vi "PICT_to_CAM.vi"(4 "Pict Refnum":refnum<vi>, 5 "IntGraph Refnum":refnum<vi>, 6 "Ny":i32, 7 "Yo":i32, 8 "Nx":i32, 9 "Xo":i32) -> (0 "Ny CAM":i16, 1 "Nx CAM":i16, 2 "Yo CAM":i16, 3 "Xo CAM":i16)   [LabVIEW 2011]
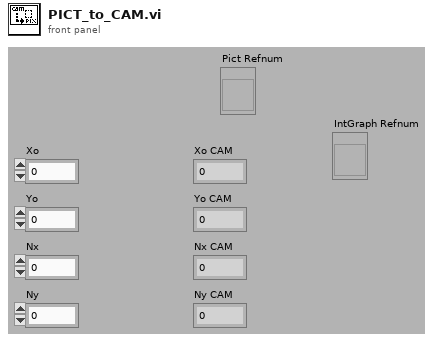
[diagram p1: front panel]
types:
  T1 = typedef "LVBoundsTypeDef.ctl" = cluster{"Width":u32, "Height":u32}
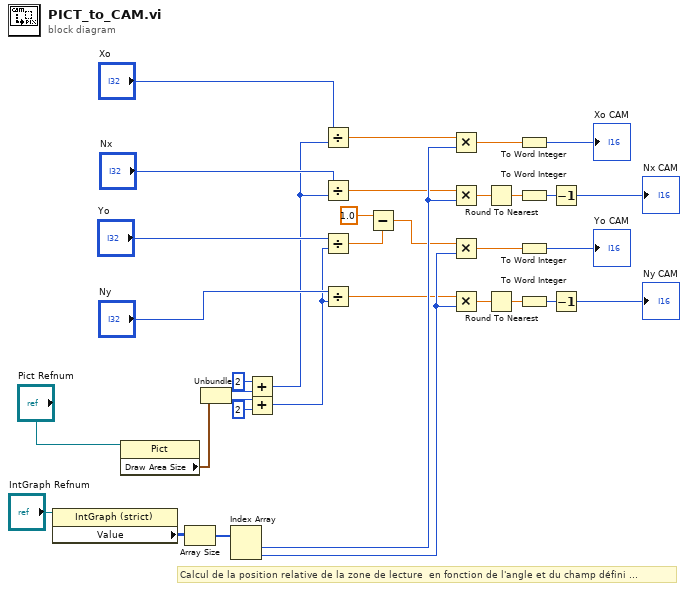
[diagram p0: block diagram]
diagram:
  # "Calcul de la position relative de la zone de lecture  en fonction de l'angle et du champ défini ..."
  n1 = property class="IntGraph (strict)"(reference="IntGraph Refnum") -> ("Value"=w28:u32[][])  [unwired: 1 in, 2 out]
  n2 = property class="Pict"(reference="Pict Refnum") -> ("Draw Area Size"=w26:T1)  [unwired: 1 in, 2 out]
  n3 = Array Size(array=w28) -> (size(s)=w25:i32[])
  n4 = Unbundle(w26) -> ("Width"=w8:u32, "Height"=w9:u32)
  n5 = Index Array(array=w25) -> (element #1=w24:i32, element #2=w23:i32)  [unwired: 2 in]
  n6 = Add(x=u32 2, y=w8) -> (x+y=w7:u32)
  n7 = Add(x=w9, y=u32 2) -> (x+y=w6:u32)
  n8 = Divide(x="Xo", y=w7) -> (x/y=w18:dbl)
  n9 = Divide(x="Nx", y=w7) -> (x/y=w17:dbl)
  n10 = Divide(x="Yo", y=w6) -> (x/y=w3:dbl)
  n11 = Divide(x="Ny", y=w6) -> (x/y=w16:dbl)
  n12 = Subtract(x=1.0, y=w3) -> (x-y=w1:dbl)
  n13 = Multiply(x=w18, y=w24) -> (x*y=w13:dbl)
  n14 = Multiply(x=w17, y=w24) -> (x*y=w34:dbl)
  n15 = Multiply(x=w1, y=w23) -> (x*y=w12:dbl)
  n16 = Multiply(x=w16, y=w23) -> (x*y=w35:dbl)
  n17 = Round To Nearest(number=w34) -> (nearest integer value=w32:dbl)
  n18 = Round To Nearest(number=w35) -> (nearest integer value=w33:dbl)
  n19 = To Word Integer(number=w13) -> (16bit integer=→"Xo CAM":i16)
  n20 = To Word Integer(number=w32) -> (16bit integer=w14:i16)
  n21 = To Word Integer(number=w12) -> (16bit integer=→"Yo CAM":i16)
  n22 = To Word Integer(number=w33) -> (16bit integer=w30:i16)
  n23 = Decrement(x=w14) -> (x-1=→"Nx CAM":i16)
  n24 = Decrement(x=w30) -> (x-1=→"Ny CAM":i16)
